vi "Post_Pro_Results_Hierarchy.vi"() -> ()   [LabVIEW 2013]
uses:
  Anemometry Sub Vis/Controls/File_Selector_Type.ctl
panel:
  out "Currently Processing":path
  out "Files to Post Process":path[](array[path])
  in  "Save results to":T1(ring)=enum."Original Results Filenames with _PP"
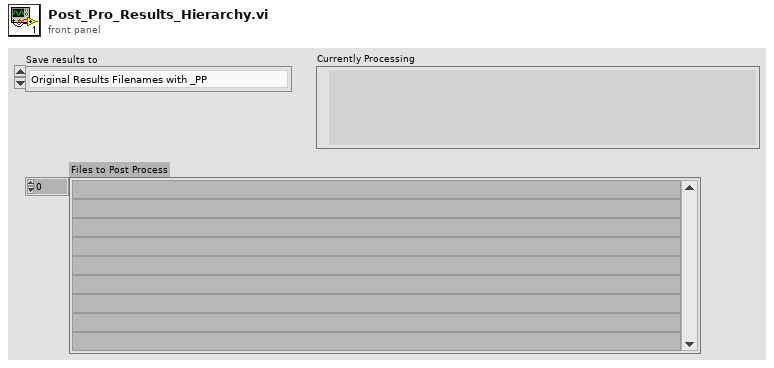
[diagram p1: front panel]
types:
  T1 = enum16{"A single file", "Original Results Filenames with _PP", "Current Results Filenames"}
  T2 = typedef "File_Selector_Type.ctl" = enum16{"The Selected File", "The Selected Folder", "Files containing the search string in the selected folder", "All files listed in selected file"}
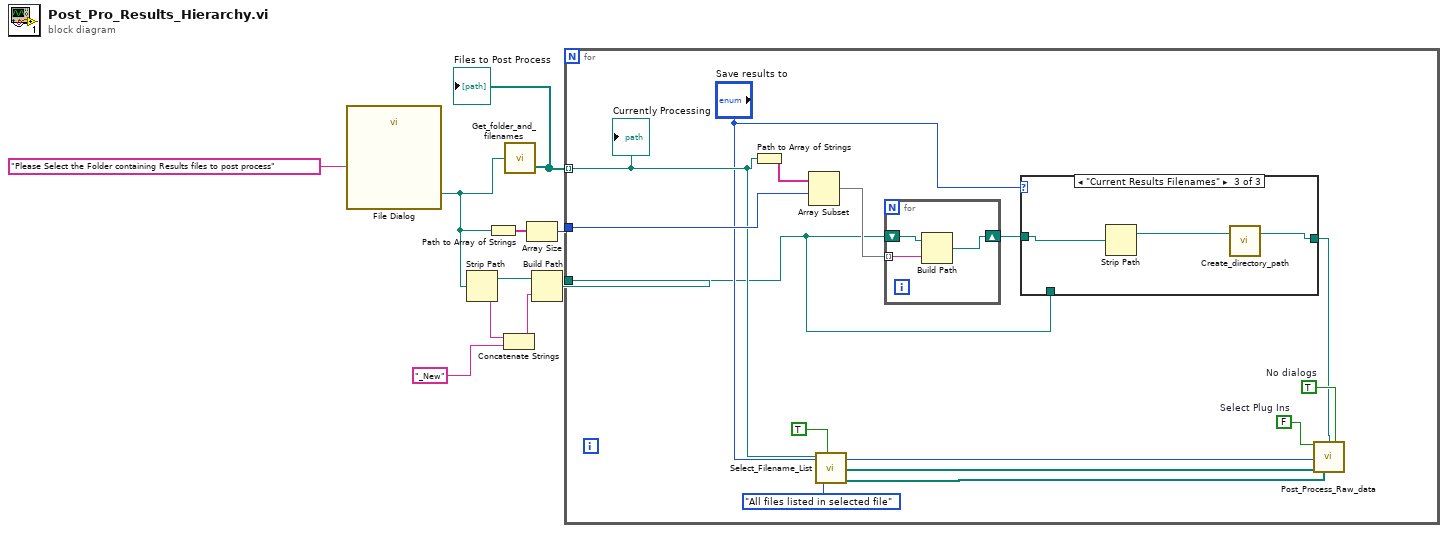
[diagram p0: block diagram]
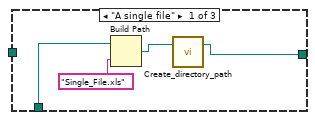
[diagram p2: hidden frame]
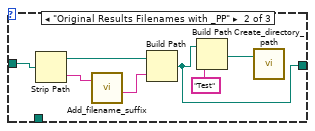
[diagram p3: hidden frame]
diagram:
  n1 = call "File Dialog"("prompt"="Please Select the Folder containing Results files to post process") -> ("selected path"=w6:path)  [unwired: 11 in, 3 out]
  n2 = Strip Path(path=w6) -> (stripped path=w5:path, name=w4:string)
  n3 = Path to Array of Strings(0:w6) -> (2:w9:string[])  [unwired: 1 out]
  n4 = Concatenate Strings(w4, "_New" ("string")) -> (w3:string)
  n5 = call "Get_folder_and_filenames.vi"("file path (dialog if empty)"=w6) -> ("Files"=w8:path[])  [unwired: 1 out]
  "Files to Post Process" <- w8
  n6 = Array Size(array=w9) -> (size(s)=w7:i32)
  n7 = Build Path(base path=w5, name or relative path=w3) -> (appended path=w1:path)
  n8 = for {
    tunnel: w8 -> [w19] mode=indexing
    tunnel: w7 -> [w23]
    tunnel: w1 -> [w12]
    w14 = TRUE  # No dialogs
    w20 = FALSE  # Select Plug Ins
    n9 = Path to Array of Strings(0:w19) -> (2:w24:string[])  [unwired: 1 out]
    n10 = Array Subset(array=w24, index=w23) -> (w22:string[])  [unwired: 1 in]
    n11 = call "Select_Filename_List.vi"("No dialogs"=TRUE, "At Dialog Prompt Post Process"=File_Selector_Type."All files listed in selected file", "Previous Choice"=w19) -> ("Current Results filenames"=w16:path[], "Selected files"=w15:path[])  [unwired: 2 in, 2 out]
    n12 = for {
      tunnel: w22 -> [w39] mode=indexing
      shift-right: [w40] -> w21
      shift-left: w12 -> [w41]
      n13 = Build Path(base path=w41, name or relative path=w39) -> (appended path=w40:path)
    }
    n14 = case shown="\"Current Results Filenames\"" "Save results to" {
      tunnel: w21 -> [_ w34 w37]
      tunnel: [w25 w29 w38] -> w11
      tunnel: w12 -> [w28 _ _]
      frame "A single file" {
        n15 = Build Path(base path=w28, name or relative path="Single_File.xls") -> (appended path=w26:path)
        n16 = call "Create_directory_path.vi"("Path name"=w26) -> ("Path name Out"=w25:path)  [unwired: 1 in, 1 out]
      }
      frame "Original Results Filenames with _PP" {
        n17 = Strip Path(path=w34) -> (stripped path=w32:path, name=w33:string)
        n18 = call "Add_filename_suffix.vi"("Filename"=w33) -> ("Base name"=w35:string)  [unwired: 1 in, 3 out]
        n19 = Build Path(base path=w32, name or relative path=w35) -> (appended path=w29:path)
        n20 = Build Path(base path=w29, name or relative path="Test") -> (appended path=w30:path)
        n21 = call "Create_directory_path.vi"("Path name"=w30) -> ()  [unwired: 1 in, 2 out]
      }
      frame "Current Results Filenames" {
        n22 = Strip Path(path=w37) -> (stripped path=w36:path)  [unwired: 1 out]
        n23 = call "Create_directory_path.vi"("Path name"=w36) -> ("Path name Out"=w38:path)  [unwired: 1 in, 1 out]
      }
    }
    n24 = call "Post_Process_Raw_data.vi"("Select Plug Ins"=w20, "Post processed Results folder"=w11, "No dialogs"=w14, "Save results to"="Save results to", "Selected files"=w15, "Current Results filenames"=w16) -> ()  [unwired: 9 in, 1 out]
    "Currently Processing" <- w19
  }
